vi "getType.vi"(8 "error in (no error)":errorcluster, 11 "BlockDiagram In":refnum<class "AbstractDiagram.lvclass">) -> (0 "error out":errorcluster, 2 "type":string, 3 "BlockDiagram Out":refnum<class "AbstractDiagram.lvclass">)   [LabVIEW 2023, in "TLC_Scripto.lvlib" / "AbstractDiagram.lvclass"]
uses:
  AbstractDiagram.lvclass
  AbstractDiagram.lvclass/AbstractDiagram.ctl
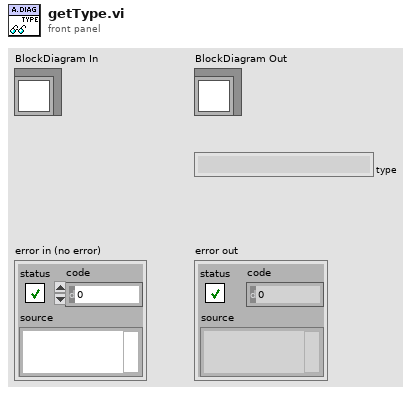
[diagram p1: front panel]
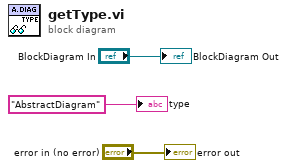
[diagram p0: block diagram]
diagram:
  "error out" <- "error in (no error)"
  "BlockDiagram Out" <- "BlockDiagram In"
  "type" <- "AbstractDiagram" ("type")
